vi "Launch Waiting Functions.vi"(8 "error in (no error)":errorcluster, 11 "Controller in":refnum<class "Controller.lvclass">) -> (0 "error out":errorcluster, 3 "Controller out":refnum<class "Controller.lvclass">)   [LabVIEW 2016, in "Controller Actor.lvlib" / "Controller.lvclass"]
uses:
  <userlib>/Common Components/Controller/Controller.lvclass
  <userlib>/Common Components/Controller/Messages/Launch Functions Message/Launch Functions Message.lvclass
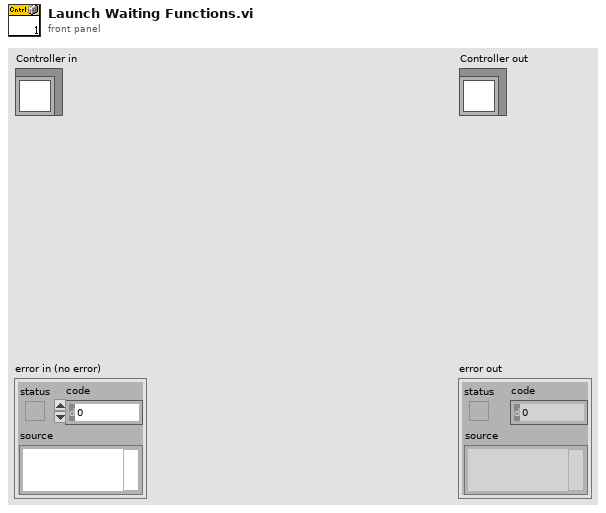
[diagram p1: front panel]
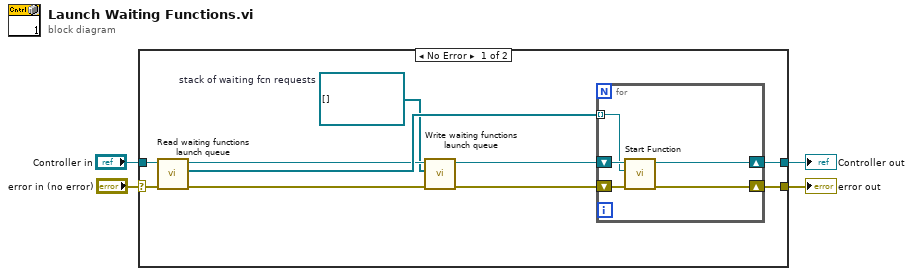
[diagram p0: block diagram]
diagram:
  n1 = case shown="No Error" "error in (no error)" {
    selector: "error in (no error)" -> [w5 w21]
    tunnel: [w12 w21] -> w3
    tunnel: [w9 w20] -> w1
    tunnel: "Controller in" -> [w14 w20]
    frame No Error {
      w6 = refnum<class "Launch Functions Message.lvclass">[] []  # stack of waiting fcn requests
      n2 = call <userlib>:"Read waiting functions launch queue.vi"("error in (no error)"=w5, "Controller in"=w14) -> ("error out"=w7:errorcluster, "stack of waiting fcn requests"=w13:refnum<class "Launch Functions Message.lvclass">[], "Controller out"=w11:refnum<class "Controller.lvclass">)  [unwired: 7 in]
      n3 = call <userlib>:"Write waiting functions launch queue.vi"("error in (no error)"=w7, "stack of waiting fcn requests"=w6, "Controller in"=w11) -> ("error out"=w8:errorcluster, "Controller out"=w10:refnum<class "Controller.lvclass">)  [unwired: 7 in]
      n4 = for {
        tunnel: w13 -> [w15] mode=indexing
        shift-right: [w18] -> w9
        shift-left: w10 -> [w19]
        shift-right: [w16] -> w12
        shift-left: w8 -> [w17]
        n5 = call-dynamic "Start Function.vi"("error in (no error)"=w17, "Launch Functions Message in"=w15, "Controller in"=w19) -> ("error out"=w16:errorcluster, "Controller out"=w18:refnum<class "Controller.lvclass">)  [unwired: 7 in]
      }
    }
    frame Error {
    }
  }
  "error out" <- w3
  "Controller out" <- w1
